vi "syringeControl.vi"(4 "syringeReverseVol":dbl, 5 "Address":u16, 6 "volume(mL)":dbl, 7 "buttonAspirate":bool, 8 "error in (no error)":errorcluster, 9 "buttonRefill":bool, 10 "buttonDispense":bool, 11 "VISA Refnum in":refnum<visa-resource-name>) -> (0 "error out":errorcluster, 3 "VISA Refnum out":refnum<visa-resource-name>)   [LabVIEW 2021]
uses:
  globalVariables.vi
  Copy of Kloehn V6 Series Folder/Copy of Kloehn V6 Series.lvlib
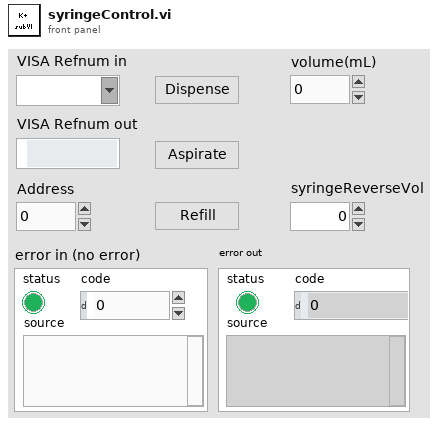
[diagram p1: front panel]
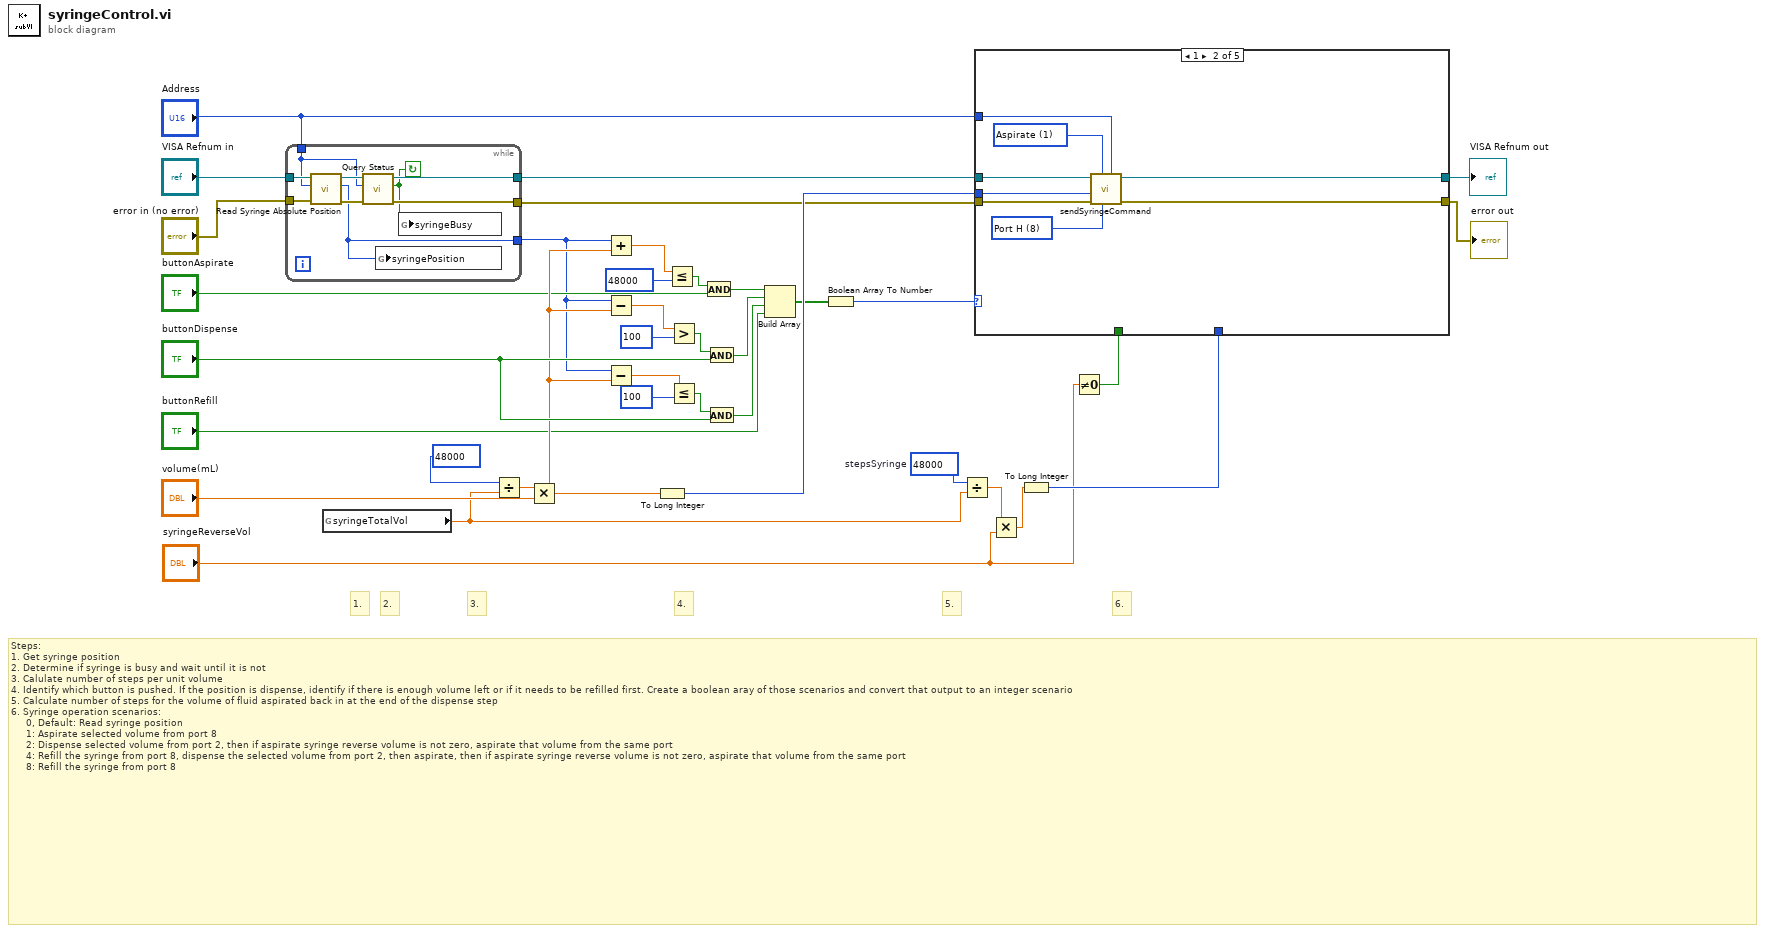
[diagram p0: block diagram]
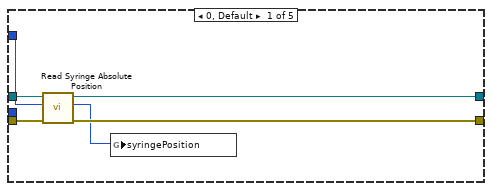
[diagram p2: hidden frame]
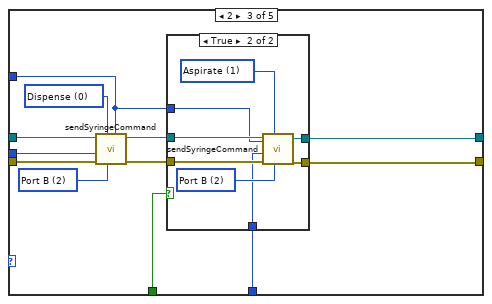
[diagram p3: hidden frame]
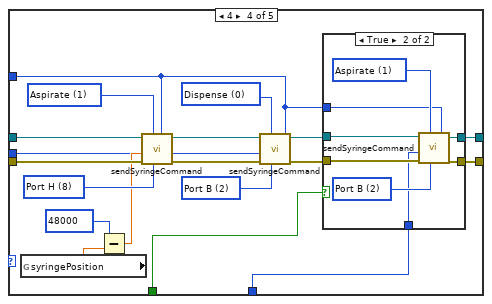
[diagram p5: hidden frame]
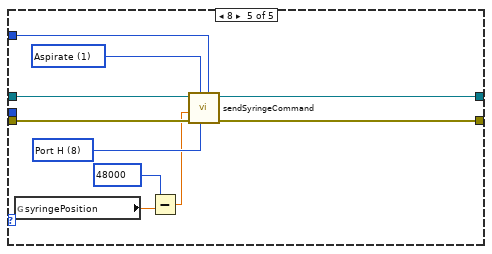
[diagram p7: hidden frame]
diagram:
  w6 = 48000  # stepsSyringe
  # "Steps:\n1. Get syringe position\n2. Determine if syringe is busy and wait until it is not\n3. Calulate number of steps per unit volume\n4. Identify which button is pushed. If the position is dispense, identify if there is enough volume left or if it needs to be refilled first. Create a boolean aray of those scenarios and convert that output to an integer scenario\n5. Calculate number of steps for the volume of fluid aspirated back in at the end of the dispense step\n6. Syringe operation scenarios:\n     0, Default: Read syringe position\n     1: Aspirate selected volume from port 8\n     2: Dispense selected volume from port 2, then if aspirate syringe reverse volume is not zero, aspirate that volume from the same port \n     4: Refill the syringe from port 8, dispense the selected volume from port 2, then aspirate, then if aspirate syringe reverse volume is not zero, aspirate that volume from the same port \n     8: Refill the syringe from port 8"
  # "6."
  # "5."
  # "4."
  # "3."
  # "2."
  # "1."
  n1 = while {
    tunnel: "VISA Refnum in" -> [w46]
    tunnel: "error in (no error)" -> [w45]
    tunnel: [w42] -> w9
    tunnel: [w41] -> w8
    tunnel: "Address" -> [w40]
    tunnel: [w38] -> w13
    stop <- w39 continue-if-true
    n2 = call "Read Syringe Absolute Position.vi"("error in (no error)"=w45, "Address (1)"=w40, "VISA resource name"=w46) -> ("error out"=w44:errorcluster, "Absolute Position"=w38:u16, "VISA resource name out"=w43:refnum<visa-resource-name>)  [unwired: 6 in]
    n3 = call "Query Status.vi"("error in (no error)"=w44, "Address (1)"=w40, "VISA resource name"=w43) -> ("error out"=w41:errorcluster, "Status"=w39:bool, "VISA resource name out"=w42:refnum<visa-resource-name>)  [unwired: 6 in]
    n4 = global write "globalVariables.vi" "syringePosition"(w38) -> ()
    n5 = global write "globalVariables.vi" "syringeBusy"(w39) -> ()
  }
  n6 = global read "globalVariables.vi" "syringeTotalVol"() -> (w2:dbl)
  n7 = Divide(x=48000, y=w2) -> (x/y=w26:dbl)
  n8 = Multiply(x=w26, y="volume(mL)") -> (x*y=w33:dbl)
  n9 = Add(x=w13, y=w33) -> (x+y=w23:dbl)
  n10 = Subtract(x=w13, y=w33) -> (x-y=w20:dbl)
  n11 = Subtract(x=w13, y=w33) -> (x-y=w32:dbl)
  n12 = To Long Integer(number=w33) -> (32bit integer=w37:i32)
  n13 = Less Or Equal?(x=w23, y=48000) -> (x <= y?=w22:bool)
  n14 = Greater?(x=w20, y=100) -> (0:w19:bool)
  n15 = Less Or Equal?(x=w32, y=100) -> (x <= y?=w31:bool)
  n16 = And(x=w22, y="buttonAspirate") -> (x .and. y?=w24:bool)
  n17 = And(x=w19, y="buttonDispense") -> (x .and. y?=w17:bool)
  n18 = And(x=w31, y="buttonDispense") -> (x .and. y?=w35:bool)
  n19 = Build Array(w24, w17, w35, "buttonRefill") -> (w28:bool[])
  n20 = Boolean Array To Number(Boolean array=w28) -> (number=w36:u32)
  n21 = Divide(x=w6, y=w2) -> (x/y=w5:dbl)
  n22 = Multiply(x=w5, y="syringeReverseVol") -> (x*y=w7:dbl)
  n23 = To Long Integer(number=w7) -> (32bit integer=w4:i32)
  n24 = Not Equal To 0?(x="syringeReverseVol") -> (x != 0?=w1:bool)
  n25 = case shown="1" w36 {
    tunnel: w9 -> [w51 w60 w72 w101 w121]
    tunnel: w8 -> [w50 w59 w71 w100 w120]
    tunnel: [w48 w57 w65 w86 w118] -> w14
    tunnel: [w49 w56 w64 w87 w117] -> w15
    tunnel: "Address" -> [w52 w55 w63 w85 w116]
    tunnel: w37 -> [_ w53 w68 w91 _]
    tunnel: w4 -> [_ _ w62 w84 _]
    tunnel: w1 -> [_ _ w61 w83 _]
    frame 0, Default {
      n26 = call "Read Syringe Absolute Position.vi"("error in (no error)"=w50, "Address (1)"=w52, "VISA resource name"=w51) -> ("error out"=w49:errorcluster, "Absolute Position"=w47:u16, "VISA resource name out"=w48:refnum<visa-resource-name>)  [unwired: 6 in]
      n27 = global write "globalVariables.vi" "syringePosition"(w47) -> ()
    }
    frame 1 {
      w54 = u16 8 items=["Port A"=1, "Port B"=2, "Port C"=3, "Port D"=4, "Port E"=5, "Port F"=6, "Port G"=7, "Port H"=8, "Port I"=9, "Port J"=10, "Port K"=11, "Port L"=12] ("Valve Position (1:Port A)")
      w58 = u16 1 items=["Dispense", "Aspirate", "Handshake Dispense"] ("Flow Direction (0: Dispense)")
      n28 = call "sendSyringeCommand.vi"("Address"=w55, "Flow Direction (0: Dispense)"=w58, "Valve Position (1:Port A)"=w54, "error in (no error)"=w59, "Number of Steps"=w53, "VISA Refnum in"=w60) -> ("syringeError"=w56:errorcluster, "VISA Refnum out"=w57:refnum<visa-resource-name>)  [unwired: 4 in]
    }
    frame 2 {
      w69 = u16 2 items=["Port A"=1, "Port B"=2, "Port C"=3, "Port D"=4, "Port E"=5, "Port F"=6, "Port G"=7, "Port H"=8, "Port I"=9, "Port J"=10, "Port K"=11, "Port L"=12] ("Valve Position (1:Port A)")
      w70 = u16 0 items=["Dispense", "Aspirate", "Handshake Dispense"] ("Flow Direction (0: Dispense)")
      n29 = call "sendSyringeCommand.vi"("Address"=w63, "Flow Direction (0: Dispense)"=w70, "Valve Position (1:Port A)"=w69, "error in (no error)"=w71, "Number of Steps"=w68, "VISA Refnum in"=w72) -> ("syringeError"=w66:errorcluster, "VISA Refnum out"=w67:refnum<visa-resource-name>)  [unwired: 4 in]
      n30 = case shown="True" w61 {
        tunnel: w67 -> [w74 w80]
        tunnel: w66 -> [w73 w79]
        tunnel: [w74 w78] -> w65
        tunnel: [w73 w77] -> w64
        tunnel: w63 -> [_ w76]
        tunnel: w62 -> [_ w75]
        frame False {
        }
        frame True {
          w81 = u16 2 items=["Port A"=1, "Port B"=2, "Port C"=3, "Port D"=4, "Port E"=5, "Port F"=6, "Port G"=7, "Port H"=8, "Port I"=9, "Port J"=10, "Port K"=11, "Port L"=12] ("Valve Position (1:Port A)")
          w82 = u16 1 items=["Dispense", "Aspirate", "Handshake Dispense"] ("Flow Direction (0: Dispense)")
          n31 = call "sendSyringeCommand.vi"("Address"=w76, "Flow Direction (0: Dispense)"=w82, "Valve Position (1:Port A)"=w81, "error in (no error)"=w79, "Number of Steps"=w75, "VISA Refnum in"=w80) -> ("syringeError"=w77:errorcluster, "VISA Refnum out"=w78:refnum<visa-resource-name>)  [unwired: 4 in]
        }
      }
    }
    frame 4 {
      w94 = u16 2 items=["Port A"=1, "Port B"=2, "Port C"=3, "Port D"=4, "Port E"=5, "Port F"=6, "Port G"=7, "Port H"=8, "Port I"=9, "Port J"=10, "Port K"=11, "Port L"=12] ("Valve Position (1:Port A)")
      w95 = u16 0 items=["Dispense", "Aspirate", "Handshake Dispense"] ("Flow Direction (0: Dispense)")
      w98 = u16 8 items=["Port A"=1, "Port B"=2, "Port C"=3, "Port D"=4, "Port E"=5, "Port F"=6, "Port G"=7, "Port H"=8, "Port I"=9, "Port J"=10, "Port K"=11, "Port L"=12] ("Valve Position (1:Port A)")
      w99 = u16 1 items=["Dispense", "Aspirate", "Handshake Dispense"] ("Flow Direction (0: Dispense)")
      n32 = global read "globalVariables.vi" "syringePosition"() -> (w90:dbl)
      n33 = Subtract(x=48000, y=w90) -> (x-y=w96:dbl)
      n34 = call "sendSyringeCommand.vi"("Address"=w85, "Flow Direction (0: Dispense)"=w99, "Valve Position (1:Port A)"=w98, "error in (no error)"=w100, "Number of Steps"=w96, "VISA Refnum in"=w101) -> ("syringeError"=w92:errorcluster, "VISA Refnum out"=w93:refnum<visa-resource-name>)  [unwired: 4 in]
      n35 = call "sendSyringeCommand.vi"("Address"=w85, "Flow Direction (0: Dispense)"=w95, "Valve Position (1:Port A)"=w94, "error in (no error)"=w92, "Number of Steps"=w91, "VISA Refnum in"=w93) -> ("syringeError"=w88:errorcluster, "VISA Refnum out"=w89:refnum<visa-resource-name>)  [unwired: 4 in]
      n36 = case shown="True" w83 {
        tunnel: w89 -> [w103 w109]
        tunnel: w88 -> [w102 w108]
        tunnel: [w103 w107] -> w86
        tunnel: [w102 w106] -> w87
        tunnel: w85 -> [_ w105]
        tunnel: w84 -> [_ w104]
        frame False {
        }
        frame True {
          w110 = u16 2 items=["Port A"=1, "Port B"=2, "Port C"=3, "Port D"=4, "Port E"=5, "Port F"=6, "Port G"=7, "Port H"=8, "Port I"=9, "Port J"=10, "Port K"=11, "Port L"=12] ("Valve Position (1:Port A)")
          w111 = u16 1 items=["Dispense", "Aspirate", "Handshake Dispense"] ("Flow Direction (0: Dispense)")
          n37 = call "sendSyringeCommand.vi"("Address"=w105, "Flow Direction (0: Dispense)"=w111, "Valve Position (1:Port A)"=w110, "error in (no error)"=w108, "Number of Steps"=w104, "VISA Refnum in"=w109) -> ("syringeError"=w106:errorcluster, "VISA Refnum out"=w107:refnum<visa-resource-name>)  [unwired: 4 in]
        }
      }
    }
    frame 8 {
      w115 = u16 8 items=["Port A"=1, "Port B"=2, "Port C"=3, "Port D"=4, "Port E"=5, "Port F"=6, "Port G"=7, "Port H"=8, "Port I"=9, "Port J"=10, "Port K"=11, "Port L"=12] ("Valve Position (1:Port A)")
      w119 = u16 1 items=["Dispense", "Aspirate", "Handshake Dispense"] ("Flow Direction (0: Dispense)")
      n38 = global read "globalVariables.vi" "syringePosition"() -> (w112:dbl)
      n39 = Subtract(x=48000, y=w112) -> (x-y=w113:dbl)
      n40 = call "sendSyringeCommand.vi"("Address"=w116, "Flow Direction (0: Dispense)"=w119, "Valve Position (1:Port A)"=w115, "error in (no error)"=w120, "Number of Steps"=w113, "VISA Refnum in"=w121) -> ("syringeError"=w117:errorcluster, "VISA Refnum out"=w118:refnum<visa-resource-name>)  [unwired: 4 in]
    }
  }
  "error out" <- w15
  "VISA Refnum out" <- w14
